vi "Init_USB_DEV_SN_To_Global.vi"() -> (1 "Number  of dev Connected":i32, 2 "USB_DEV_2":string, 3 "USB_DEV_1":string, 4 "USB_DEV_4":string, 5 "USB_DEV_3":string)   [LabVIEW 2015]
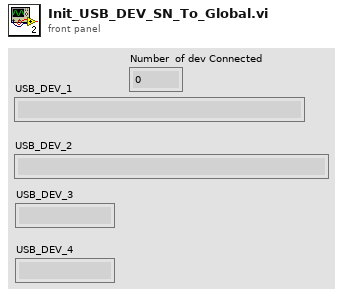
[diagram p1: front panel]
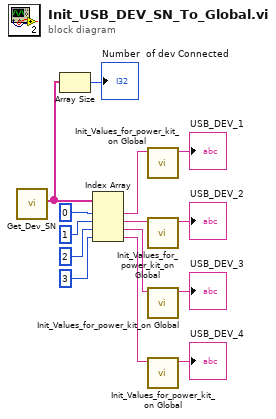
[diagram p0: block diagram]
diagram:
  n1 = call "Get_Dev_SN.vi"() -> ("Dev_SN 2"=w8:string[])  [unwired: 8 in, 3 out]
  n2 = Array Size(array=w8) -> (size(s)=→"Number  of dev Connected":i32)
  n3 = Index Array(array=w8, index #1=0 ("index"), index #2=1 ("index"), index #3=2 ("index"), index #4=3 ("index")) -> (element #1=w13:string, element #2=w10:string, element #3=w4:string, element #4=w1:string)
  n4 = call "Init_Values_for_power_kit_on Global.vi"("DevSerialNum"=w13) -> ("JSON string"=→"USB_DEV_1":string)  [unwired: 10 in]
  n5 = call "Init_Values_for_power_kit_on Global.vi"("DevSerialNum"=w10) -> ("JSON string"=→"USB_DEV_2":string)  [unwired: 10 in]
  n6 = call "Init_Values_for_power_kit_on Global.vi"("DevSerialNum"=w4) -> ("JSON string"=→"USB_DEV_3":string)  [unwired: 10 in]
  n7 = call "Init_Values_for_power_kit_on Global.vi"("DevSerialNum"=w1) -> ("JSON string"=→"USB_DEV_4":string)  [unwired: 10 in]
